vi "Set inOpen.vi"(8 "error in (no error)":errorcluster, 10 "inOpen":bool, 11 "AbstractDstarNode in":refnum<class "NI_Robotics_AbstractDstarNode.lvclass">) -> (0 "error out":errorcluster, 3 "AbstractDstarNode out":refnum<class "NI_Robotics_AbstractDstarNode.lvclass">)   [LabVIEW 2017, in "NI_Robotics_AbstractDstarNode.lvclass"]
uses:
  <vilib>/robotics/Navigation/shared/MapNode/AbstractDstarNode/NI_Robotics_AbstractDstarNode.lvclass
  <vilib>/robotics/Navigation/shared/MapNode/AbstractDstarNode/NI_Robotics_AbstractDstarNode.lvclass/NI_Robotics_AbstractDstarNode.ctl
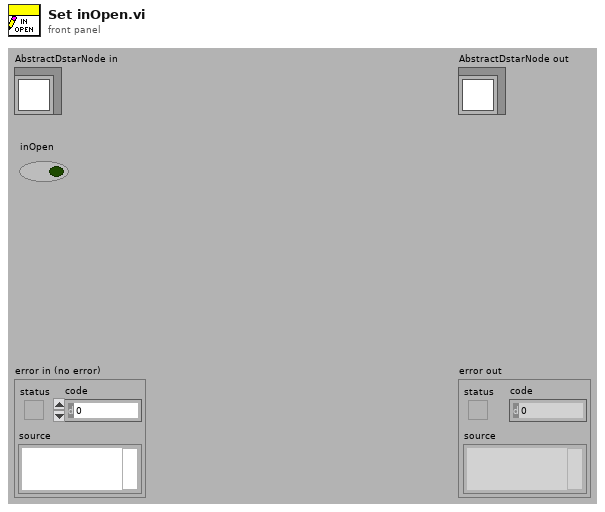
[diagram p1: front panel]
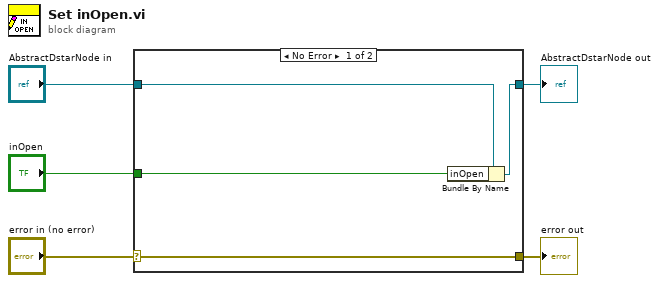
[diagram p0: block diagram]
diagram:
  n1 = case shown="No Error" "error in (no error)" {
    selector: "error in (no error)" -> [w9 w10]
    tunnel: [w9 w10] -> w4
    tunnel: [w7 w11] -> w2
    tunnel: "AbstractDstarNode in" -> [w8 w11]
    tunnel: "inOpen" -> [w6 _]
    frame No Error {
      n2 = Bundle By Name(cluster=w8, "inOpen"=w6) -> (w7:refnum<class "NI_Robotics_AbstractDstarNode.lvclass">)
    }
    frame Error {
    }
  }
  "error out" <- w4
  "AbstractDstarNode out" <- w2
